vi "Finish.vi"(8 "error in (no error)":errorcluster, 11 "Process In":refnum<class "Process.lvclass">) -> (0 "error out":errorcluster, 3 "Process Out":refnum<class "Process.lvclass">)   [LabVIEW 2020, in "Process.lvclass"]
uses:
  Process.lvclass
  C:/git/astemes-triarc-framework/source/Framework/Logging/Logging.lvclass
  C:/git/astemes-triarc-framework/source/Framework/Base/Base.lvclass
  Public/Lifecycle/Lifecycle State.ctl
  Process.lvclass/Process.ctl
  Logging/Logging.lvclass
  C:/git/astemes-triarc-framework/source/Framework/Process/Process.lvclass
  C:/git/astemes-triarc-framework/source/Framework/Error Handler Interface/Error Handler Interface.lvclass
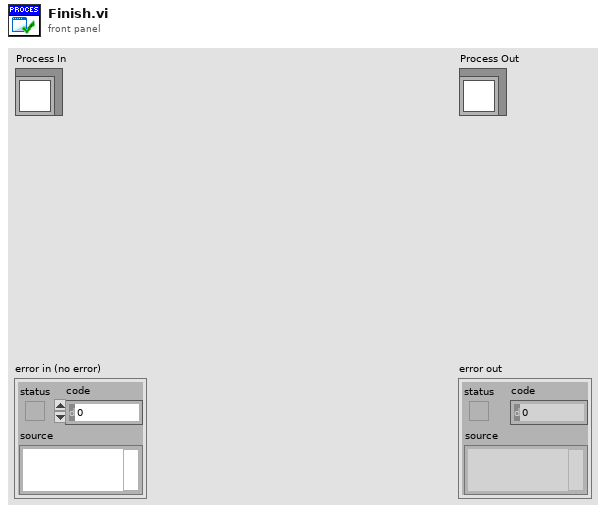
[diagram p1: front panel]
types:
  T1 = typedef "Process.lvclass/Lifecycle State.ctl" = enum16{"Uninitialized", "Initialized", "Started", "Running", "Stopped", "Finished"}
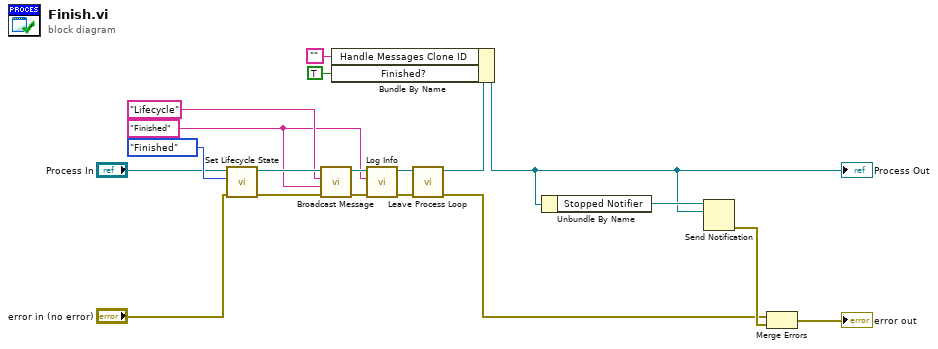
[diagram p0: block diagram]
diagram:
  w5 = "Finished" ("Message")
  n1 = call "Set Lifecycle State.vi"("error in (no error)"="error in (no error)", "Lifecycle State"=Lifecycle_State."Finished", "Process In"="Process In") -> ("error out"=w16:errorcluster, "Process Out"=w17:refnum<class "Process.lvclass">)  [unwired: 7 in]
  n2 = call-dynamic "Broadcast Message.vi"("error in (no error)"=w16, "Message Data"=w5, "Message"="Lifecycle", "Process In"=w17) -> ("error out"=w10:errorcluster, "Process Out"=w6:refnum<class "Process.lvclass">)  [unwired: 6 in]
  n3 = call "Log Info.vi"("error in (no error)"=w10, "Message"=w5, "Logging In"=w6) -> ("error out"=w9:errorcluster, "Logging Out"=w2:refnum<class "Process.lvclass">)  [unwired: 7 in]
  n4 = call "Leave Process Loop.vi"("error in (no error)"=w9, "Process In"=w2) -> ("error out"=w3:errorcluster, "Process Out"=w1:refnum<class "Process.lvclass">)  [unwired: 8 in]
  n5 = Bundle By Name(cluster=w1, "Handle Messages Clone ID"="", "Finished?"=TRUE) -> (w8:refnum<class "Process.lvclass">)
  "Process Out" <- w8
  n6 = Unbundle By Name(w8) -> ("Stopped Notifier"=w19:refnum<notifier>)
  n7 = Send Notification(notification=w8, notifier=w19) -> (error out=w13:errorcluster)  [unwired: 1 in, 1 out]
  n8 = Merge Errors(w3, w13) -> (→"error out":errorcluster)
